vi "ADIS16448 Scale Data.vi"(8 "error in (no error)":errorcluster, 10 "New Data In":u8[](array[numeric])) -> (0 "error out":errorcluster, 1 "Data Good?":bool, 2 "Data Out":dbl[](array[numeric]))   [LabVIEW 2019]
panel:
  out "Calculated CRC-16":u16
  out "Received CRC-16":u16
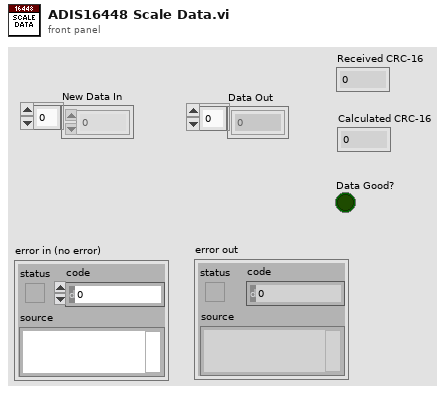
[diagram p1: front panel]
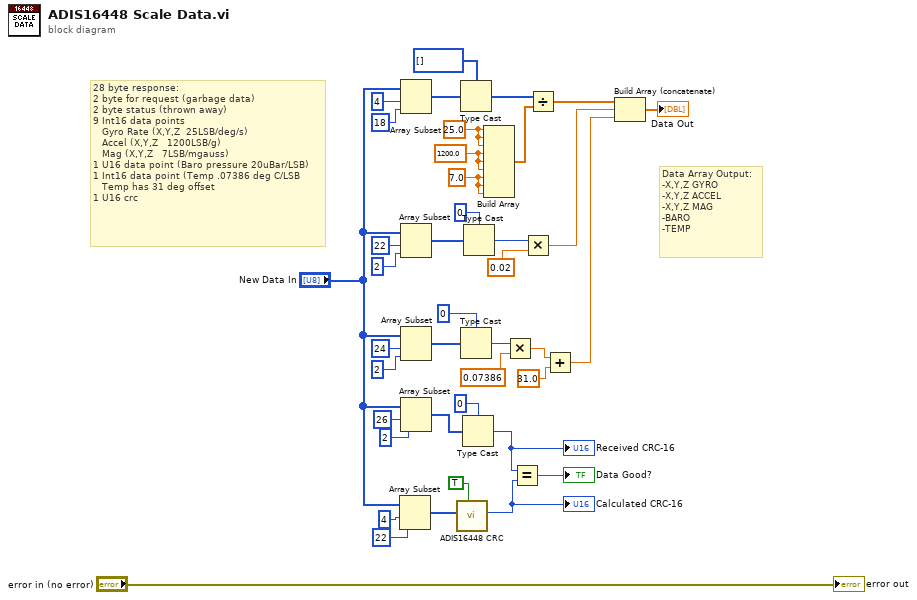
[diagram p0: block diagram]
diagram:
  w38 = 7.0
  w39 = 1200.0
  w40 = 25.0 ("element")
  # "Data Array Output:\n-X,Y,Z GYRO\n-X,Y,Z ACCEL\n-X,Y,Z MAG\n-BARO\n-TEMP"
  # "28 byte response:\n2 byte for request (garbage data)\n2 byte status (thrown away)\n9 Int16 data points\n   Gyro Rate (X,Y,Z  25LSB/deg/s)\n   Accel (X,Y,Z   1200LSB/g)\n   Mag (X,Y,Z   7LSB/mgauss)\n1 U16 data point (Baro pressure 20uBar/LSB)\n1 Int16 data point (Temp .07386 deg C/LSB\n   Temp has 31 deg offset\n1 U16 crc"
  n1 = Array Subset(array="New Data In", index=4, length=22) -> (w6:u8[])
  n2 = Array Subset(array="New Data In", index=4, length=18) -> (w18:u8[])
  n3 = Array Subset(array="New Data In", index=22, length=2) -> (w24:u8[])
  n4 = Array Subset(array="New Data In", index=24, length=2) -> (w22:u8[])
  n5 = Array Subset(array="New Data In", index=26, length=2) -> (w12:u8[])
  n6 = call "ADIS16448 CRC.vi"("Look-Up Table Method?"=TRUE, "Byte Array (MSB-First)"=w6) -> ("CRC16-ADIS"=w5:u16)  [unwired: 9 in]
  "Calculated CRC-16" <- w5
  n7 = Type Cast(type=i16[] [], x=w18) -> (*(type *) &x=w17:i16[])
  n8 = Type Cast(type=i16 0, x=w22) -> (*(type *) &x=w19:i16)
  n9 = Type Cast(type=u16 0, x=w12) -> (*(type *) &x=w9:u16)
  "Received CRC-16" <- w9
  n10 = Type Cast(type=u16 0, x=w24) -> (*(type *) &x=w20:u16)
  n11 = Build Array(w40, w40, w40, w39, w39, w39, w38, w38, w38) -> (w37:dbl[])
  n12 = Multiply(x=w19, y=0.07386 ("element")) -> (x*y=w34:dbl)
  n13 = Equal?(x=w9, y=w5) -> (x = y?=→"Data Good?":bool)
  n14 = Multiply(x=w20, y=0.02) -> (x*y=w31:dbl)
  n15 = Divide(x=w17, y=w37) -> (x/y=w3:dbl[])
  n16 = Add(x=w34, y=31.0) -> (x+y=w32:dbl)
  n17 = Build Array (concatenate)(w3, w31, w32) -> (→"Data Out":dbl[])
  "error out" <- "error in (no error)"
